vi "Get TIC graph.vi"(8 "error in":errorcluster, 10 "Array":i64[][](array[numeric]), 11 "Byte Stream File in":refnum<file>) -> (0 "error out":errorcluster, 2 "Cluster":cluster{dbl[], u32[]}, 3 "Byte Stream File out":refnum<file>)   [LabVIEW 2015]
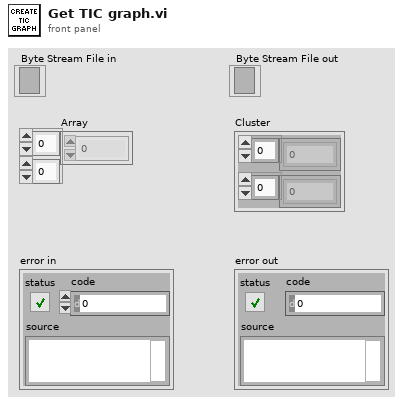
[diagram p1: front panel]
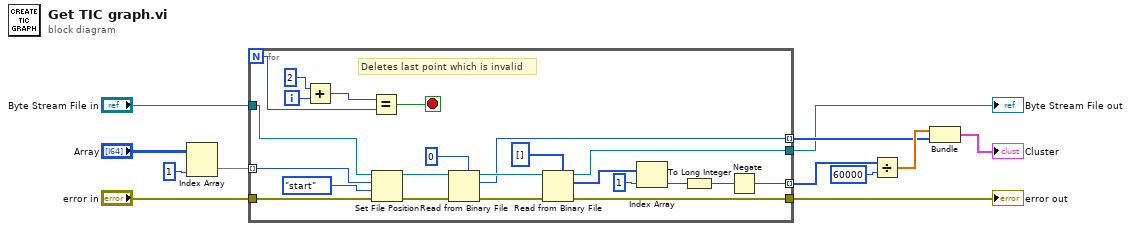
[diagram p0: block diagram]
diagram:
  n1 = Index Array(array="Array", index (col)=1 ("disabled index (col)")) -> (element=w5:i64[])  [unwired: 1 in]
  n2 = for {
    N -> [w19]
    tunnel: w5 -> [w32] mode=indexing
    tunnel: "Byte Stream File in" -> [w31]
    tunnel: [w29] -> w7
    tunnel: [w24] -> w11 mode=indexing
    tunnel: [w23] -> w8 mode=indexing
    tunnel: "error in" -> [w16]
    tunnel: [w13] -> w1
    i -> [w21]
    stop <- w17 stop-if-true
    # "Deletes last point which is invalid"
    n3 = Add(x=2, y=w21) -> (x+y=w18:i32)
    n4 = Equal?(x=w18, y=w19) -> (x = y?=w17:bool)
    n5 = Set File Position(offset (in bytes) (0)=w32, refnum=w31, from (0:start)=enum16{"start", "end", "current"}."start" ("pos mode (0:2)"), error in=w16) -> (refnum out=w34:refnum<file>, error out=w15:errorcluster)
    n6 = Read from Binary File(5:u32 0, 8:w15, 11:w34) -> (0:w14:errorcluster, 2:w23:u32, 3:w30:refnum<file>)  [unwired: 4 out]
    n7 = Read from Binary File(5:u32[] [] ("Spectrum"), 8:w14, 11:w30) -> (0:w13:errorcluster, 2:w22:u32[], 3:w29:refnum<file>)  [unwired: 4 out]
    n8 = Index Array(array=w22, index=1) -> (element=w28:u32)
    n9 = To Long Integer(number=w28) -> (32bit integer=w26:i32)
    n10 = Negate(x=w26) -> (-x=w24:i32)
  }
  "Byte Stream File out" <- w7
  "error out" <- w1
  n11 = Divide(x=w11, y=60000 ("index")) -> (x/y=w10:dbl[])
  n12 = Bundle(w10, w8) -> (→"Cluster":cluster{dbl[], u32[]})  [unwired: 1 in]
